vi "toml_api_load.vi"(7 "resolved path":path, 8 "error in (no error)":errorcluster, 10 "operation":T1(ring), 11 "vi in":refnum<vi>) -> (0 "error out":errorcluster, 2 "file reloaded":bool, 3 "vi out":refnum<vi>)   [LabVIEW 2017]
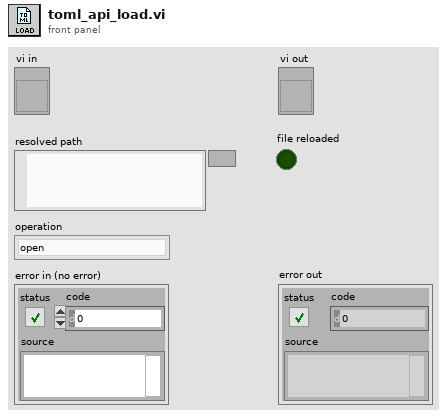
[diagram p1: front panel]
types:
  T1 = enum16{"open", "replace", "create", "open or create", "replace or create", "replace or create with confirmation"}
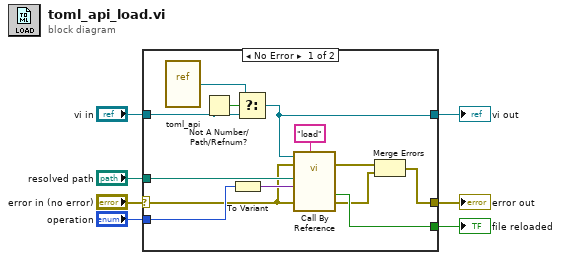
[diagram p0: block diagram]
diagram:
  n1 = case shown="No Error" "error in (no error)" {
    selector: "error in (no error)" -> [w10 w22]
    tunnel: "operation" -> [w19 _]
    tunnel: [w18 _] -> w6
    tunnel: "resolved path" -> [w16 _]
    tunnel: [w12 w22] -> w4
    tunnel: "vi in" -> [w9 w21]
    tunnel: [w8 w21] -> w1
    frame No Error {
      n2 = vi-ref "toml_api.vi"() -> (w15:refnum<vi>)
      n3 = Not A Number/Path/Refnum?(number/path/refnum=w9) -> (NaN/Path/Refnum?=w14:bool)
      n4 = To Variant(anything=w19) -> (Variant=w20:variant)
      n5 = Select(t=w15, s=w14, f=w9) -> (s? t:f=w8:refnum<vi>)
      n6 = call-by-ref "?"(reference=w8, error in=w10, "cmd"="load", 8:"error in (no error)"=w10, "data in"=w20, "path in"=w16) -> (error out=w11:errorcluster, 0:"error out"=w17:errorcluster, "return"=w18:bool)  [unwired: 4 in, 3 out]
      n7 = Merge Errors(w11, w17) -> (w12:errorcluster)
    }
    frame Error {
    }
  }
  "file reloaded" <- w6
  "error out" <- w4
  "vi out" <- w1
